vi "XPS_DelayLine_Move.vi"() -> ()   [LabVIEW 2025]
uses:
  C:/Users/user/Nutstore/1/Nutstore/fs-TA/Library/Newport.XPS.CommandInterface.dll
  Library/Newport.XPS.CommandInterface.dll
panel:
  in  "Num of Scans":i32=5
  out "error out":errorcluster
  out "XPS Reference":refnum<k24>
  in  "Group Name":string="Group2"
  in  "MaximumTjerkTime":dbl=0.05 format="%#_13g"
  in  "MinimumTjerkTime":dbl=0.005 format="%#_13g"
  in  "Acceleration":dbl=50.0 format="%#_13g"
  in  "Velocity":dbl=50.0 format="%#_13g"
  in  "Positioner Name":string="Group2.Pos"
  in  "Target Position":dbl[](array[numeric])=[100.0, 200.0, 300.0]
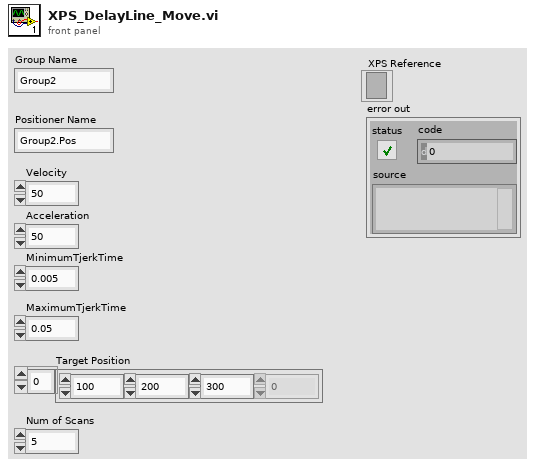
[diagram p1: front panel]
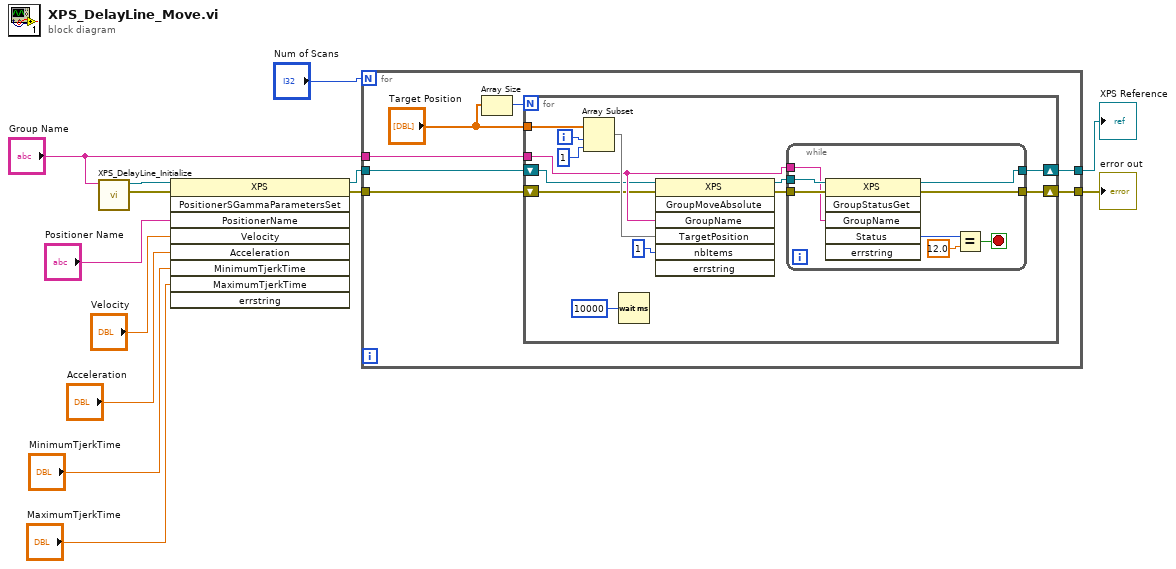
[diagram p0: block diagram]
diagram:
  n1 = call "XPS_DelayLine_Initialize.vi"("Group Name"="Group Name") -> ("XPS Error"=w11:errorcluster, "XPS Reference"=w12:refnum<k24>)  [unwired: 9 in]
  n2 = invoke class="XPS" method="PositionerSGammaParametersSet"(reference=w12, error in=w11, "PositionerName"="Positioner Name", "Velocity"="Velocity", "Acceleration"="Acceleration", "MinimumTjerkTime"="MinimumTjerkTime", "MaximumTjerkTime"="MaximumTjerkTime") -> (reference out=w10:refnum<k24>, error out=w9:errorcluster)  [unwired: 2 in, 7 out]
  n3 = for {
    N: "Num of Scans" -> [_]
    tunnel: "Group Name" -> [w18]
    tunnel: w10 -> [w17]
    tunnel: w9 -> [w16]
    tunnel: [w15] -> w3
    tunnel: [w14] -> w2
    n4 = Array Size(array="Target Position") -> (size(s)=w19:i32)
    n5 = for {
      N: w19 -> [_]
      tunnel: "Target Position" -> [w32]
      tunnel: w18 -> [w28]
      shift-right: [w22] -> w15
      shift-left: w16 -> [w26]
      shift-right: [w23] -> w14
      shift-left: w17 -> [w27]
      i -> [w33]
      n6 = Array Subset(array=w32, index=w33, length=1) -> (w30:dbl[])
      n7 = Wait (ms)(milliseconds to wait=u32 10000) -> ()  [unwired: 1 out]
      n8 = invoke class="XPS" method="GroupMoveAbsolute"(reference=w27, error in=w26, "GroupName"=w28, "TargetPosition"=w30, "nbItems"=1) -> (reference out=w25:refnum<k24>, error out=w24:errorcluster)  [unwired: 2 in, 5 out]
      n9 = while {
        tunnel: w28 -> [w34]
        tunnel: w25 -> [w39]
        tunnel: w24 -> [w38]
        tunnel: [w37] -> w23
        tunnel: [w36] -> w22
        stop <- w41 stop-if-true
        n10 = invoke class="XPS" method="GroupStatusGet"(reference=w39, error in=w38, "GroupName"=w34) -> (reference out=w37:refnum<k24>, error out=w36:errorcluster, "Status"=w35:i32)  [unwired: 3 in, 3 out]
        n11 = Equal?(x=w35, y=12.0) -> (x = y?=w41:bool)
      }
    }
  }
  "error out" <- w3
  "XPS Reference" <- w2
